vi "3.2.2_BOOST_Power_Tune.vi"(6 "Data in":T1, 8 "error in (no error)":errorcluster, 9 "AllControls In":T2, 10 "?":T3, 11 "Message Queue out":T4) -> (0 "error out":errorcluster, 1 "Flow":string, 2 "Data":T3, 3 "Message Queue Out":T4, 4 "Data out":T1)   [LabVIEW 2017]
uses:
  Depends/AMC/subVIs/TypeDefs/amc_Message Queue.ctl
  Depends/AMC/subVIs/TypeDefs/amc_Message.ctl
  Depends/Tools/Keyed Array/Tools_KeyedArray KeyedArray.ctl
  Ctrls/Data.ctl
  Ctrls/CSV_Data.ctl
  Ctrls/AllControls.ctl
  DIPC 692 Daemon API/typdef/get_parameter.ctl
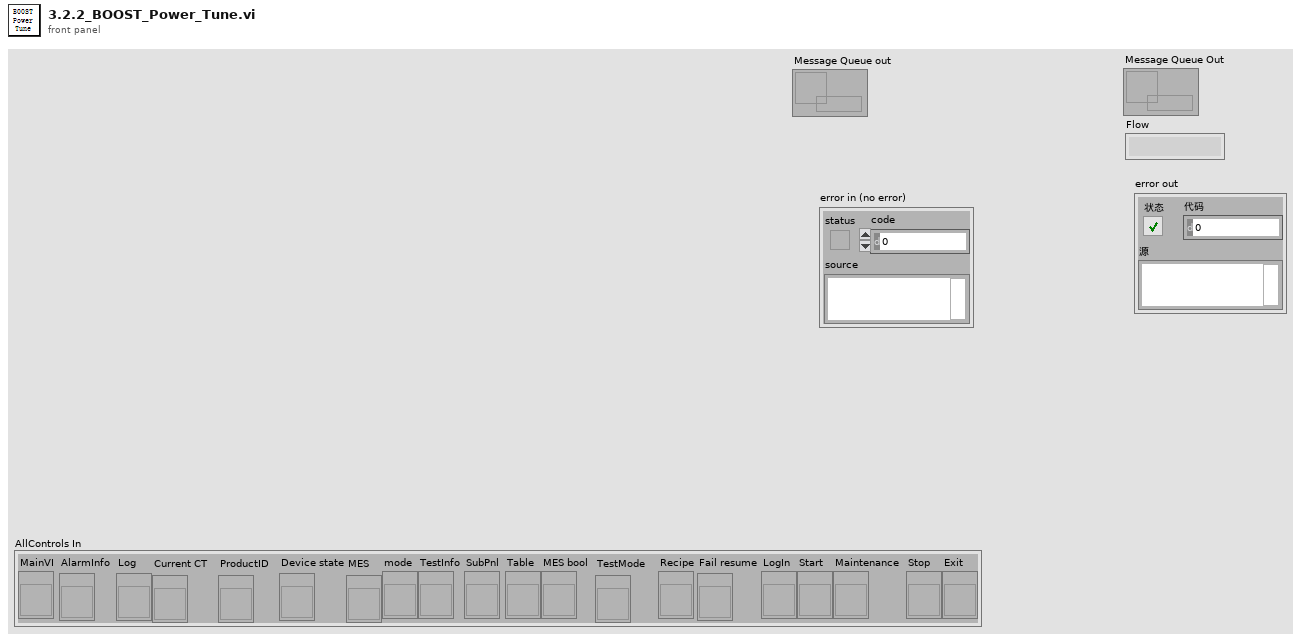
[diagram p1: front panel]
types:
  T1 = typedef "CSV_Data.ctl" = cluster{"Initialisation":cluster{"LMT - Connect UUT (con COM)":string, "LMT - Software Version (rrel)":string, "LMT - Write SKU file (wskuc)":string, "LMT - SKU file name":string, "Connect UUT DDM":string, "Read DDM EOL Timestamp - Mode":string, "Read DDM EOL Timestamp - Timestamp":string, "Read DDM EOL Timestamp - Rig ID":string, "Read DDM EOL Timestamp - Passmark ID":string, "Read DDM EOL Timestamp - Passmark Rev":string, "Software Version before flashing":string, "Read Hardware Serial":string, "UUT DDM SN":string, "Compare DDM SN with MES SN":string, "Backup PCBA Calibration EEPROM Response - CAL":string, "Flash Firmware Version":string, "Check SW Version":string, "Read DDM SW Version after flashing":string, "Set SKU Config":string, "Ready Status":string, "Set Device Mode to EOL":string, "DDM Parameter - Voltage":string, "DDM Parameter - Current":string, "DDM Parameter - Power":string, "DDM Parameter - Speed":string, "DDM Parameter - Pressure":string, "Tester Parameter - Voltage":string, "Tester Parameter - Current":string, "Tester Parameter - Power":string, "Tester Parameter - Ambient Pressure":string, "Tester Parameter - Ambient Temperature":string, "Calculated Parameter - DDM Pressure Corrected":string, "Calculated Parameter - DDM Real Power":string, "Calculated Parameter - Delta V":string}, "BEMF_Calibration":cluster{"Calibration Result - eol_cold_bemf_temp":string, "DDM Ambient Temp":string, "Restriction Plate Diameter":string, "Calibration Result - eol_bemf_mp_cold_coef_a":string, "Calibration Result - eol_bemf_mp_cold_coef_b":string, "Calibration Result - eol_bemf_mp_cold_coef_c":string, "Calibration Result - eol_bemf_lsi_cold_ref_coeffs":string, "Get - Calibration Result - eol_bemf_lsi_speed":string, "Get - Calibration Result - eol_bemf_lsi_integral_0":string, "Calibration Result - eol_bemf_lsi_integral_1":string, "Get - Calibration Result - eol_bemf_lsi_integral_2":string, "Get - Calibration Result - eol_cold_bemf":string, "Get - Calibration Result - eol_cold_bemf_fisf":string, "Finalise Calibration":string, "Compare -Calibration Result - eol_cold_bemf":string, "Compare -Calibration Result - eol_cold_bemf_fisf":string}, "ECO":cluster{"Reset Power Tune":string, "Reset BEMF FISF Calibration":string, "Restriction Plate Diameter":string, "ECO - Stabilisation Time":string, "ECO - DDM Parameter - Voltage":string, "ECO - DDM Parameter - Current":string, "ECO - DDM Parameter - Power":string, "ECO - DDM Parameter - Measured Power":string, "ECO - DDM Parameter - Speed":string, "ECO - DDM Parameter - Pressure":string, "ECO - Tester Parameter - Voltage":string, "ECO - Tester Parameter - Current":string, "ECO - Tester Parameter - Power":string, "ECO - Tester Parameter - Ambient Pressure":string, "ECO - Tester Parameter - Ambient Temperature":string, "ECO - Tester Parameter - Ambient Humidity":string, "ECO - Calculated Parameter - DDM Pressure Corrected":string, "ECO - Calculated Parameter - DDM Real Power":string, "ECO - Calculated Parameter - Delta V":string, "ECO - Calculated Parameter - Flowrate":string, "ECO - Calculated Parameter - Airwatt":string, "ECO - Formula":string, "PT ECO - Power Tune Mode Status":string}, "BOOST":cluster{"Restriction Plate Diameter":string, "BOOST - Stabilisation Time":string, "BOOST - DDM Parameter - Voltage":string, "BOOST - DDM Parameter - Current":string, "BOOST - DDM Parameter - Power":string, "BOOST - DDM Parameter - Measured Power":string, "BOOST - DDM Parameter - Speed":string, "BOOST - DDM Parameter - Pressure":string, "BOOST - Tester Parameter - Voltage":string, "BOOST - Tester Parameter - Current":string, "BOOST - Tester Parameter - Power":string, "BOOST - Tester Parameter - Ambient Pressure":string, "BOOST - Tester Parameter - Ambient Temperature":string, "BOOST - Tester Parameter - Ambient Humidity":string, "BOOST - Calculated Parameter - DDM Pressure Corrected":string, "BOOST - Calculated Parameter - DDM Real Power":string, "BOOST - Calculated Parameter - Delta V":string, "BOOST - Calculated Parameter - Flowrate":string, "BOOST - Calculated Parameter - Airwatt":string, "BOOST - Get AM Presence":string, "Air Muscle Turn Off Status":string, "BOOST - Air Muscle Calculated Parameter - Airwatt B":string, "BOOST - Air Muscle Calculate Airwatt Delta":string, "PT BOOST - Power Tune Mode Status":string, "Finalise Calibration":string, "ECO - Get AW Calibration value":string, "BOOST - Get AW Calibration value":string}, "MAX":cluster{"Restriction Plate Diameter":string, "MAX - Stabilisation Time":string, "Get Average Delta Tmag (LSIdelta_FISFdelta_LSItmag_FISFtmag_IIRtmag)":string, "Get Average Delta Tmag FISF":string, "MAX - DDM Parameter - Voltage":string, "MAX - DDM Parameter - Current":string, "MAX - DDM Parameter - Power":string, "MAX - DDM Parameter - Measured Power":string, "MAX - DDM Parameter - Speed":string, "MAX - DDM Parameter - Pressure":string, "MAX - Tester Parameter - Voltage":string, "MAX - Tester Parameter - Current":string, "MAX - Tester Parameter - Power":string, "MAX - Tester Parameter - Ambient Pressure":string, "MAX - Tester Parameter - Ambient Temperature":string, "MAX - Tester Parameter - Ambient Humidity":string, "MAX - Calculated Parameter - DDM Pressure Corrected":string, "MAX - Calculated Parameter - DDM Real Power":string, "MAX - Calculated Parameter - Delta V":string, "MAX - Calculated Parameter - Flowrate":string, "MAX - Calculated Parameter - Airwatt":string, "MAX_FISF_Check_Average_Delta_Tmag":string, "MAX - FISF - BEMF Finetune Result":string, "MAX tune - Delta P1":string, "MAX tune - Calculated Parameter - Airwatt":string, "Calculate Delta Airwatts - MAX finetune - Delta P2":string, "MAX finetune - DDM Parameter - Voltage":string, "MAX finetune - DDM Parameter - Current":string, "MAX finetune - DDM Parameter - Power":string, "MAX finetune - DDM Parameter - Measured Power":string, "MAX finetune - DDM Parameter - Speed":string, "MAX finetune - DDM Parameter - Pressure":string, "MAX finetune - Tester Parameter - Voltage":string, "MAX finetune - Tester Parameter - Current":string, "MAX finetune - Tester Parameter - Power":string, "MAX finetune - Tester Parameter - Ambient Pressure":string, "MAX finetune - Tester Parameter - Ambient Temperature":string, "MAX finetune - Tester Parameter - Ambient Humidity":string, "MAX finetune - Calculated Parameter - DDM Pressure Corrected":string, "MAX finetune - Calculated Parameter - DDM Real Power":string, "MAX finetune - Calculated Parameter - Delta V":string, "MAX finetune - Calculated Parameter - Flowrate":string, "MAX finetune - Calculated Parameter - Airwatt":string, "Check Derate Result":string, "Delta Tmag FISF":string, "Get Hot BEMF Result":string, "Calculate delta Pressure":string, "Finalise Calibration":string, "Calculate & Check Delta BEMF":string, "Delta P Airwatts Value":string}, "LL":cluster{"DDM Ambient Temp":string, "Restriction Plate Diameter":string, "LL - DDM Parameter - Voltage":string, "LL - DDM Parameter - Current":string, "LL - DDM Parameter - Power":string, "LL - DDM Parameter - Measured Power":string, "LL - DDM Parameter - Speed":string, "LL - DDM Parameter - Pressure":string, "LL - Tester Parameter - Voltage":string, "LL - Tester Parameter - Current":string, "LL - Tester Parameter - Power":string, "LL - DDM Real Power":string, "LL - Calibrate Task Detect LL":string}, "HL":cluster{"HL - DDM Parameter - Voltage":string, "HL - DDM Parameter - Current":string, "HL - DDM Parameter - Power":string, "HL - DDM Parameter - Measured Power":string, "HL - DDM Parameter - Speed":string, "HL - DDM Parameter - Pressure":string, "HL - Tester Parameter - Voltage":string, "HL - Tester Parameter - Current":string, "HL - Tester Parameter - Power":string, "HL - DDM Real Power":string, "HL - Calibrate Task Detect HL":string}, "LH":cluster{"Restriction Plate Diameter":string, "LH - DDM Parameter - Voltage":string, "LH - DDM Parameter - Current":string, "LH - DDM Parameter - Power":string, "LH - DDM Parameter - Measured Power":string, "LH - DDM Parameter - Speed":string, "LH - DDM Parameter - Pressure":string, "LH - Tester Parameter - Voltage":string, "LH - Tester Parameter - Current":string, "LH - Tester Parameter - Power":string, "LH - DDM Real Power":string, "LH - Calibrate Task Detect LH":string}, "HH":cluster{"HH - DDM Parameter - Voltage":string, "HH - DDM Parameter - Current":string, "HH - DDM Parameter - Power":string, "HH - DDM Parameter - Measured Power":string, "HH - DDM Parameter - Speed":string, "HH - DDM Parameter - Pressure":string, "HH - Tester Parameter - Voltage":string, "HH - Tester Parameter - Current":string, "HH - Tester Parameter - Power":string, "HH - DDM Real Power":string, "HH - Calibrate Task Detect HH":string}, "Inlet Blockage Calibration":cluster{"Inlet Blockage Calibration - DDM Parameter - Voltage":string, "Inlet Blockage Calibration - DDM Parameter - Current":string, "Inlet Blockage Calibration - DDM Parameter - Power":string, "Inlet Blockage Calibration - DDM Parameter - Measured Power":string, "Inlet Blockage Calibration - DDM Parameter - Speed":string, "Inlet Blockage Calibration - DDM Parameter - Pressure":string, "Inlet Blockage Calibration - Tester Parameter - Voltage":string, "Inlet Blockage Calibration - Tester Parameter - Current":string, "Inlet Blockage Calibration - Tester Parameter - Power":string, "Inlet Blockage Calibration - DDM Real Power":string, "Calibration Inlet Blockage_E":string, "Finalise Calibration":string, "Get Task Detect LL":string, "Get Task Detect HL":string, "Get Task Detect LH":string, "Get Task Detect HH":string, "Calibration Inlet Blockage":string, "Calibration eol cold bemf temp":string}, "GOOD":cluster{"GOOD UNIT - Clear EEPROM Error Log":string, "GOOD UNIT - Write Product Timestamp - Mode":string, "GOOD UNIT - Write Product Timestamp - Timestamp":string, "GOOD UNIT - Write Product Timestamp - Rig ID":string, "GOOD UNIT - Write Product Timestamp - Passmark ID":string, "GOOD UNIT - Write Product Timestamp - Passmark Rev":string, "GOOD UNIT - Set Device Mode to PROD":string, "GOOD UNIT - Backup PCBA Calibration EEPROM Response":string, "GOOD UNIT - Check Security Bit":string, "GOOD UNIT - Set Calibration Lock":string, "GOOD UNIT - Get_Calibration_Lock":string, "GOOD UNIT - Disconnect UUT":string}, "NG":cluster{"NG UNIT - Read NVM Error":string, "NG UNIT - Set Device Mode to FCT":string, "NG UNIT - Backup PCBA Calibration EEPROM Response - CAL":string, "NG UNIT - Backup PCBA Calibration EEPROM Response - ERROR":string, "NG UNIT - Backup PCBA Calibration EEPROM Response - USAGE":string, "NG UNIT - Disconnect UUT":string}, "SN":string, "Table":string[][], "Count":cluster{"Total":i32, "OK":i32, "NG":i32, "Yield":dbl}, "Start Time":timestamp, "daemon reference":refnum<k5>, "CT":dbl, "Config":string[][], "OK/NG":bool, "Station ID":string, "MES DDM SN":string, "MES PCBA SN":string, "Retest":string, "Lux":string, "Initialisation_Status":cluster{"LMT - Connect UUT (con COM)":string, "LMT - Software Version (rrel)":string, "LMT - Write SKU file (wskuc)":string, "LMT - SKU file name":string, "Connect UUT DDM":string, "Read DDM EOL Timestamp - Mode":string, "Read DDM EOL Timestamp - Timestamp":string, "Read DDM EOL Timestamp - Rig ID":string, "Read DDM EOL Timestamp - Passmark ID":string, "Read DDM EOL Timestamp - Passmark Rev":string, "Software Version before flashing":string, "Read Hardware Serial":string, "UUT DDM SN":string, "Compare DDM SN with MES SN":string, "Backup PCBA Calibration EEPROM Response - CAL":string, "Flash Firmware Version":string, "Check SW Version":string, "Read DDM SW Version after flashing":string, "Set SKU Config":string, "Ready Status":string, "Set Device Mode to EOL":string, "DDM Parameter - Voltage":string, "DDM Parameter - Current":string, "DDM Parameter - Power":string, "DDM Parameter - Speed":string, "DDM Parameter - Pressure":string, "Tester Parameter - Voltage":string, "Tester Parameter - Current":string, "Tester Parameter - Power":string, "Tester Parameter - Ambient Pressure":string, "Tester Parameter - Ambient Temperature":string, "Calculated Parameter - DDM Pressure Corrected":string, "Calculated Parameter - DDM Real Power":string, "Calculated Parameter - Delta V":string}, "BEMF_Calibration_Status":cluster{"Calibration Result - eol_cold_bemf_temp":string, "DDM Ambient Temp":string, "Restriction Plate Diameter":string, "Calibration Result - eol_bemf_mp_cold_coef_a":string, "Calibration Result - eol_bemf_mp_cold_coef_b":string, "Calibration Result - eol_bemf_mp_cold_coef_c":string, "Calibration Result - eol_bemf_lsi_cold_ref_coeffs":string, "Get - Calibration Result - eol_bemf_lsi_speed":string, "Get - Calibration Result - eol_bemf_lsi_integral_0":string, "Calibration Result - eol_bemf_lsi_integral_1":string, "Get - Calibration Result - eol_bemf_lsi_integral_2":string, "Get - Calibration Result - eol_cold_bemf":string, "Get - Calibration Result - eol_cold_bemf_fisf":string, "Finalise Calibration":string, "Compare -Calibration Result - eol_cold_bemf":string, "Compare -Calibration Result - eol_cold_bemf_fisf":string}, "ECO_Status":cluster{"Reset Power Tune":string, "Reset BEMF FISF Calibration":string, "Restriction Plate Diameter":string, "ECO - Stabilisation Time":string, "ECO - DDM Parameter - Voltage":string, "ECO - DDM Parameter - Current":string, "ECO - DDM Parameter - Power":string, "ECO - DDM Parameter - Measured Power":string, "ECO - DDM Parameter - Speed":string, "ECO - DDM Parameter - Pressure":string, "ECO - Tester Parameter - Voltage":string, "ECO - Tester Parameter - Current":string, "ECO - Tester Parameter - Power":string, "ECO - Tester Parameter - Ambient Pressure":string, "ECO - Tester Parameter - Ambient Temperature":string, "ECO - Tester Parameter - Ambient Humidity":string, "ECO - Calculated Parameter - DDM Pressure Corrected":string, "ECO - Calculated Parameter - DDM Real Power":string, "ECO - Calculated Parameter - Delta V":string, "ECO - Calculated Parameter - Flowrate":string, "ECO - Calculated Parameter - Airwatt":string, "ECO - Formula":string, "PT ECO - Power Tune Mode Status":string}, "BOOST_Status":cluster{"Restriction Plate Diameter":string, "BOOST - Stabilisation Time":string, "BOOST - DDM Parameter - Voltage":string, "BOOST - DDM Parameter - Current":string, "BOOST - DDM Parameter - Power":string, "BOOST - DDM Parameter - Measured Power":string, "BOOST - DDM Parameter - Speed":string, "BOOST - DDM Parameter - Pressure":string, "BOOST - Tester Parameter - Voltage":string, "BOOST - Tester Parameter - Current":string, "BOOST - Tester Parameter - Power":string, "BOOST - Tester Parameter - Ambient Pressure":string, "BOOST - Tester Parameter - Ambient Temperature":string, "BOOST - Tester Parameter - Ambient Humidity":string, "BOOST - Calculated Parameter - DDM Pressure Corrected":string, "BOOST - Calculated Parameter - DDM Real Power":string, "BOOST - Calculated Parameter - Delta V":string, "BOOST - Calculated Parameter - Flowrate":string, "BOOST - Calculated Parameter - Airwatt":string, "BOOST - Get AM Presence":string, "Air Muscle Turn Off Status":string, "BOOST - Air Muscle Calculated Parameter - Airwatt B":string, "BOOST - Air Muscle Calculate Airwatt Delta":string, "PT BOOST - Power Tune Mode Status":string, "Finalise Calibration":string, "ECO - Get AW Calibration value":string, "BOOST - Get AW Calibration value":string}, "MAX_Status":cluster{"Restriction Plate Diameter":string, "MAX - Stabilisation Time":string, "Get Average Delta Tmag (LSIdelta_FISFdelta_LSItmag_FISFtmag_IIRtmag)":string, "Get Average Delta Tmag FISF":string, "MAX - DDM Parameter - Voltage":string, "MAX - DDM Parameter - Current":string, "MAX - DDM Parameter - Power":string, "MAX - DDM Parameter - Measured Power":string, "MAX - DDM Parameter - Speed":string, "MAX - DDM Parameter - Pressure":string, "MAX - Tester Parameter - Voltage":string, "MAX - Tester Parameter - Current":string, "MAX - Tester Parameter - Power":string, "MAX - Tester Parameter - Ambient Pressure":string, "MAX - Tester Parameter - Ambient Temperature":string, "MAX - Tester Parameter - Ambient Humidity":string, "MAX - Calculated Parameter - DDM Pressure Corrected":string, "MAX - Calculated Parameter - DDM Real Power":string, "MAX - Calculated Parameter - Delta V":string, "MAX - Calculated Parameter - Flowrate":string, "MAX - Calculated Parameter - Airwatt":string, "MAX_FISF_Check_Average_Delta_Tmag":string, "MAX - FISF - BEMF Finetune Result":string, "MAX tune - Delta P1":string, "MAX tune - Calculated Parameter - Airwatt":string, "Calculate Delta Airwatts - MAX finetune - Delta P2":string, "MAX finetune - DDM Parameter - Voltage":string, "MAX finetune - DDM Parameter - Current":string, "MAX finetune - DDM Parameter - Power":string, "MAX finetune - DDM Parameter - Measured Power":string, "MAX finetune - DDM Parameter - Speed":string, "MAX finetune - DDM Parameter - Pressure":string, "MAX finetune - Tester Parameter - Voltage":string, "MAX finetune - Tester Parameter - Current":string, "MAX finetune - Tester Parameter - Power":string, "MAX finetune - Tester Parameter - Ambient Pressure":string, "MAX finetune - Tester Parameter - Ambient Temperature":string, "MAX finetune - Tester Parameter - Ambient Humidity":string, "MAX finetune - Calculated Parameter - DDM Pressure Corrected":string, "MAX finetune - Calculated Parameter - DDM Real Power":string, "MAX finetune - Calculated Parameter - Delta V":string, "MAX finetune - Calculated Parameter - Flowrate":string, "MAX finetune - Calculated Parameter - Airwatt":string, "Check Derate Result":string, "Delta Tmag FISF":string, "Get Hot BEMF Result":string, "Calculate delta Pressure":string, "Finalise Calibration":string, "Calculate & Check Delta BEMF":string, "Delta P Airwatts Value":string}, "LL_Status":cluster{"DDM Ambient Temp":string, "Restriction Plate Diameter":string, "LL - DDM Parameter - Voltage":string, "LL - DDM Parameter - Current":string, "LL - DDM Parameter - Power":string, "LL - DDM Parameter - Measured Power":string, "LL - DDM Parameter - Speed":string, "LL - DDM Parameter - Pressure":string, "LL - Tester Parameter - Voltage":string, "LL - Tester Parameter - Current":string, "LL - Tester Parameter - Power":string, "LL - DDM Real Power":string, "LL - Calibrate Task Detect LL":string}, "HL_Status":cluster{"HL - DDM Parameter - Voltage":string, "HL - DDM Parameter - Current":string, "HL - DDM Parameter - Power":string, "HL - DDM Parameter - Measured Power":string, "HL - DDM Parameter - Speed":string, "HL - DDM Parameter - Pressure":string, "HL - Tester Parameter - Voltage":string, "HL - Tester Parameter - Current":string, "HL - Tester Parameter - Power":string, "HL - DDM Real Power":string, "HL - Calibrate Task Detect HL":string}, "LH_Status":cluster{"Restriction Plate Diameter":string, "LH - DDM Parameter - Voltage":string, "LH - DDM Parameter - Current":string, "LH - DDM Parameter - Power":string, "LH - DDM Parameter - Measured Power":string, "LH - DDM Parameter - Speed":string, "LH - DDM Parameter - Pressure":string, "LH - Tester Parameter - Voltage":string, "LH - Tester Parameter - Current":string, "LH - Tester Parameter - Power":string, "LH - DDM Real Power":string, "LH - Calibrate Task Detect LH":string}, "HH_Status":cluster{"HH - DDM Parameter - Voltage":string, "HH - DDM Parameter - Current":string, "HH - DDM Parameter - Power":string, "HH - DDM Parameter - Measured Power":string, "HH - DDM Parameter - Speed":string, "HH - DDM Parameter - Pressure":string, "HH - Tester Parameter - Voltage":string, "HH - Tester Parameter - Current":string, "HH - Tester Parameter - Power":string, "HH - DDM Real Power":string, "HH - Calibrate Task Detect HH":string}, "Inlet Blockage Calibration_Status":cluster{"Inlet Blockage Calibration - DDM Parameter - Voltage":string, "Inlet Blockage Calibration - DDM Parameter - Current":string, "Inlet Blockage Calibration - DDM Parameter - Power":string, "Inlet Blockage Calibration - DDM Parameter - Measured Power":string, "Inlet Blockage Calibration - DDM Parameter - Speed":string, "Inlet Blockage Calibration - DDM Parameter - Pressure":string, "Inlet Blockage Calibration - Tester Parameter - Voltage":string, "Inlet Blockage Calibration - Tester Parameter - Current":string, "Inlet Blockage Calibration - Tester Parameter - Power":string, "Inlet Blockage Calibration - DDM Real Power":string, "Calibration Inlet Blockage_E":string, "Finalise Calibration":string, "Get Task Detect LL":string, "Get Task Detect HL":string, "Get Task Detect LH":string, "Get Task Detect HH":string, "Calibration Inlet Blockage":string, "Calibration eol cold bemf temp":string}, "GOOD_Status":cluster{"GOOD UNIT - Clear EEPROM Error Log":string, "GOOD UNIT - Write Product Timestamp - Mode":string, "GOOD UNIT - Write Product Timestamp - Timestamp":string, "GOOD UNIT - Write Product Timestamp - Rig ID":string, "GOOD UNIT - Write Product Timestamp - Passmark ID":string, "GOOD UNIT - Write Product Timestamp - Passmark Rev":string, "GOOD UNIT - Set Device Mode to PROD":string, "GOOD UNIT - Backup PCBA Calibration EEPROM Response":string, "GOOD UNIT - Check Security Bit":string, "GOOD UNIT - Set Calibration Lock":string, "GOOD UNIT - Get_Calibration_Lock":string, "GOOD UNIT - Disconnect UUT":string}, "NG_Status":cluster{"NG UNIT - Read NVM Error":string, "NG UNIT - Set Device Mode to FCT":string, "NG UNIT - Backup PCBA Calibration EEPROM Response - CAL":string, "NG UNIT - Backup PCBA Calibration EEPROM Response - ERROR":string, "NG UNIT - Backup PCBA Calibration EEPROM Response - USAGE":string, "NG UNIT - Disconnect UUT":string}, "SKU":string, "Plate_Diameter":string, "Alarm":string}
  T2 = typedef "AllControls.ctl" = cluster{"MainVI":refnum<vi>, "AlarmInfo":refnum<vi>, "Log":refnum<vi>, "Current CT":refnum<vi>, "ProductID":refnum<vi>, "Device state":refnum<vi>, "MES":refnum<vi>, "mode":refnum<vi>, "TestInfo":refnum<vi>, "SubPnl":refnum<vi>, "Table":refnum<vi>, "MES bool":refnum<vi>, "TestMode":refnum<vi>, "Recipe":refnum<vi>, "Fail resume":refnum<vi>, "LogIn":refnum<vi>, "Start":refnum<vi>, "Maintenance":refnum<vi>, "Stop":refnum<vi>, "Exit":refnum<vi>}
  T3 = typedef "Data.ctl" = cluster{"Initialisation":cluster{"DDM_Parameter":dbl[], "DDM_Parameter_status":bool[], "Get_Tester_Parameter":dbl[], "Get_Tester_Parameter_status":bool[], "Cal_Tester_Parameter":dbl[], "Cal_Tester_Parameter_status":bool[], "sw_version_before_status":bool, "sw_version_after_status":bool, "Set_SKU_Config_With_LMT_status":bool, "FCT_timestamp_status":bool, "LMT_Connect_to_UUT_status":bool}, "BEMF_Calibration":cluster{"Read_ambient_temperature":dbl, "Calibration_Vaule":dbl[], "Calibration_Vaule _B":dbl[], "Calibration_Vaule_status":bool[], "Calibration_Vaule_B_status":bool[]}, "ECO":cluster{"DDM_Parameter":dbl[], "DDM_Parameter_status":bool[], "Get_Tester_Parameter":dbl[], "Get_Tester_Parameter_status":bool[], "Cal_Tester_Parameter":dbl[], "Cal_Tester_Parameter_status":bool[], "DDM_Parameter_after_power_tune":dbl[], "Get_Tester_Parameter_after_power_tune":dbl[], "Cal_Tester_Parameter_after_power_tune":dbl[], "Cal_Tester_Parameter_after_power_tune_status":bool[], "Delta_P":dbl}, "BOOST":cluster{"DDM_Parameter":dbl[], "DDM_Parameter_status":bool[], "Get_Tester_Parameter":dbl[], "Get_Tester_Parameter_status":bool[], "Cal_Tester_Parameter":dbl[], "Cal_Tester_Parameter_status":bool[], "DDM_Parameter_after_power_tune":dbl[], "Get_Tester_Parameter_after_power_tune":dbl[], "Cal_Tester_Parameter_after_power_tune":dbl[], "Cal_Tester_Parameter_after_power_tune_status":bool[], "airwatts_am_off":dbl, "AW_Delta_(AM_on_and_off)":dbl, "AW_Delta_(AM_on_and_off)_Status":bool, "Delta_P":dbl}, "MAX":cluster{"Average_Tmag_Data":cluster{"LSI Delta in degC":dbl, "FISF Delta in degc":dbl, "LSI Tmag in degC":dbl, "Fisf Tmag in degC":dbl, "IIR Tmag in degC":dbl}, "DDM_Parameter":dbl[], "DDM_Parameter_status":bool[], "Get_Tester_Parameter":dbl[], "Get_Tester_Parameter_status":bool[], "Cal_Tester_Parameter":dbl[], "BEMF_Finetune":cluster{"eol_bemf_mp_cold_coef_c":dbl, "eol_cold_bemf_fisf_offset":dbl}, "AW_Tune":cluster{"delta_P1":dbl, "delta_P_Setting":dbl}, "DDM_Parameter_after_Airwatts_Tune":dbl[], "Get_Tester_Parameter_after_Airwatts_Tune":dbl[], "Cal_Tester_Parameter_after_Airwatts_Tune":dbl[], "DDM_Parameter_after_Airwatts_Finetune":dbl[], "Get_Tester_Parameter_after_Airwatts_Finetune":dbl[], "Cal_Tester_Parameter_after_Airwatts_Finetune":dbl[], "AW_Finetune":cluster{"delta_P2":dbl, "delta_P_Setting":dbl}, "Delta_Tmag_after_tune":cluster{"LSI Delta in degC":dbl, "FISF Delta in degc":dbl, "LSI Tmag in degC":dbl, "Fisf Tmag in degC":dbl, "IIR Tmag in degC":dbl}, "Hot Bemf in mV":dbl, "DDM_Pressure":dbl, "Delta_Pressure":dbl, " Cold Bemf in mV":dbl, " delta Bemf":dbl, " delta p":dbl, "Delta_Pressure_status":bool, " delta Bemf_status":bool, "LSI Delta in degC_status":bool, "FISF Delta in degc_status":bool, "Max_check_derate_status_status":bool, "Average_All_data":dbl[][], "Average_Tmag_Data_status":bool[], "Average_Tmag_Data_after_tune_status":bool[], "Cal_Tester_Parameter_status":bool[], "Cal_Tester_Parameter_status_after_Airwatts_Tune":bool[], "Cal_Tester_Parameter_status_after_Airwatts_FineTune":bool[]}, "Task_Detect_Calib":cluster{"LL":cluster{"DDM_Parameter":dbl[], "DDM_Parameter_status":bool[], "Get_Tester_Parameter":dbl[], "Get_Tester_Parameter_status":bool[], "Set_task_detect_A":dbl, "Set_task_detect_A_Status":bool}, "HL":cluster{"DDM_Parameter":dbl[], "DDM_Parameter_status":bool[], "Get_Tester_Parameter":dbl[], "Get_Tester_Parameter_status":bool[], "Set_task_detect_B":dbl, "Set_task_detect_B_Status":bool}, "LH":cluster{"DDM_Parameter":dbl[], "DDM_Parameter_status":bool[], "Get_Tester_Parameter":dbl[], "Get_Tester_Parameter_status":bool[], "Set_task_detect_C":dbl, "Set_task_detect_C_Status":bool}, "HH":cluster{"DDM_Parameter":dbl[], "DDM_Parameter_status":bool[], "Get_Tester_Parameter":dbl[], "Get_Tester_Parameter_status":bool[], "Set_task_detect_D":dbl, "Read_and_check_calibration_Status":bool[], "Set_task_detect_D_Status":bool}, "Get_eol_inlet_blockage_E":dbl, "Calib_vaule":cluster{"Get_task_detect_LL":dbl, "Get_task_detect_HL":dbl, "Get_task_detect_LH":dbl, "Get_task_detect_HH":dbl, "eol_inlet_blockage":dbl, "eol_code_bemf_temp":dbl}, "calibrated temp":dbl, "Inlet_Blockage_Calibration":cluster{"DDM_Parameter":dbl[], "DDM_Parameter_status":bool[], "Get_Tester_Parameter":dbl[], "Get_Tester_Parameter_status":bool[]}, "Get_eol_inlet_blockage_E_Status":bool}, "good":cluster{"Write_Product_TS":cluster{"TIMESTAMP":i64, "RIG_ID":i64, "PASSMARK_ID":i64, "PASSMARK_REV":i64}, "Read_Product_TS":cluster{"TIMESTAMP":i64, "RIG_ID":i64, "PASSMARK_ID":i64, "PASSMARK_REV":i64}, "Good_Check_Secuity_Bit_Stauts":bool}}
  T4 = typedef "amc_Message Queue.ctl" = refnum<queue>
  T5 = typedef "HD Config.ctl" = cluster{" PC":cluster{"PC Address":u8[], "PC Port":i32}, "FCO":cluster{"COM":refnum<visa-resource-name>, "Baudrate":u32}, "DC Power ":cluster{"COM":refnum<visa-resource-name>, "Baudrate":u32}, "PW3336":cluster{"COM":refnum<visa-resource-name>, "Baudrate":u32}, "Lefoo":cluster{"COM":refnum<visa-resource-name>, "Baudrate":u32}, "Tempt&Hum":cluster{"COM":refnum<visa-resource-name>, "Baudrate":u32}, "DIPC":cluster{"COM":refnum<visa-resource-name>}, "Daemon":cluster{"IP Address":string, "Port":u16, "Retry":u16}, "NFC":cluster{"COM":refnum<visa-resource-name>, "Baudrate":u32}, "Fail_resume_mode":bool, "GRR":bool}
  T6 = typedef "get_parameter.ctl" = string
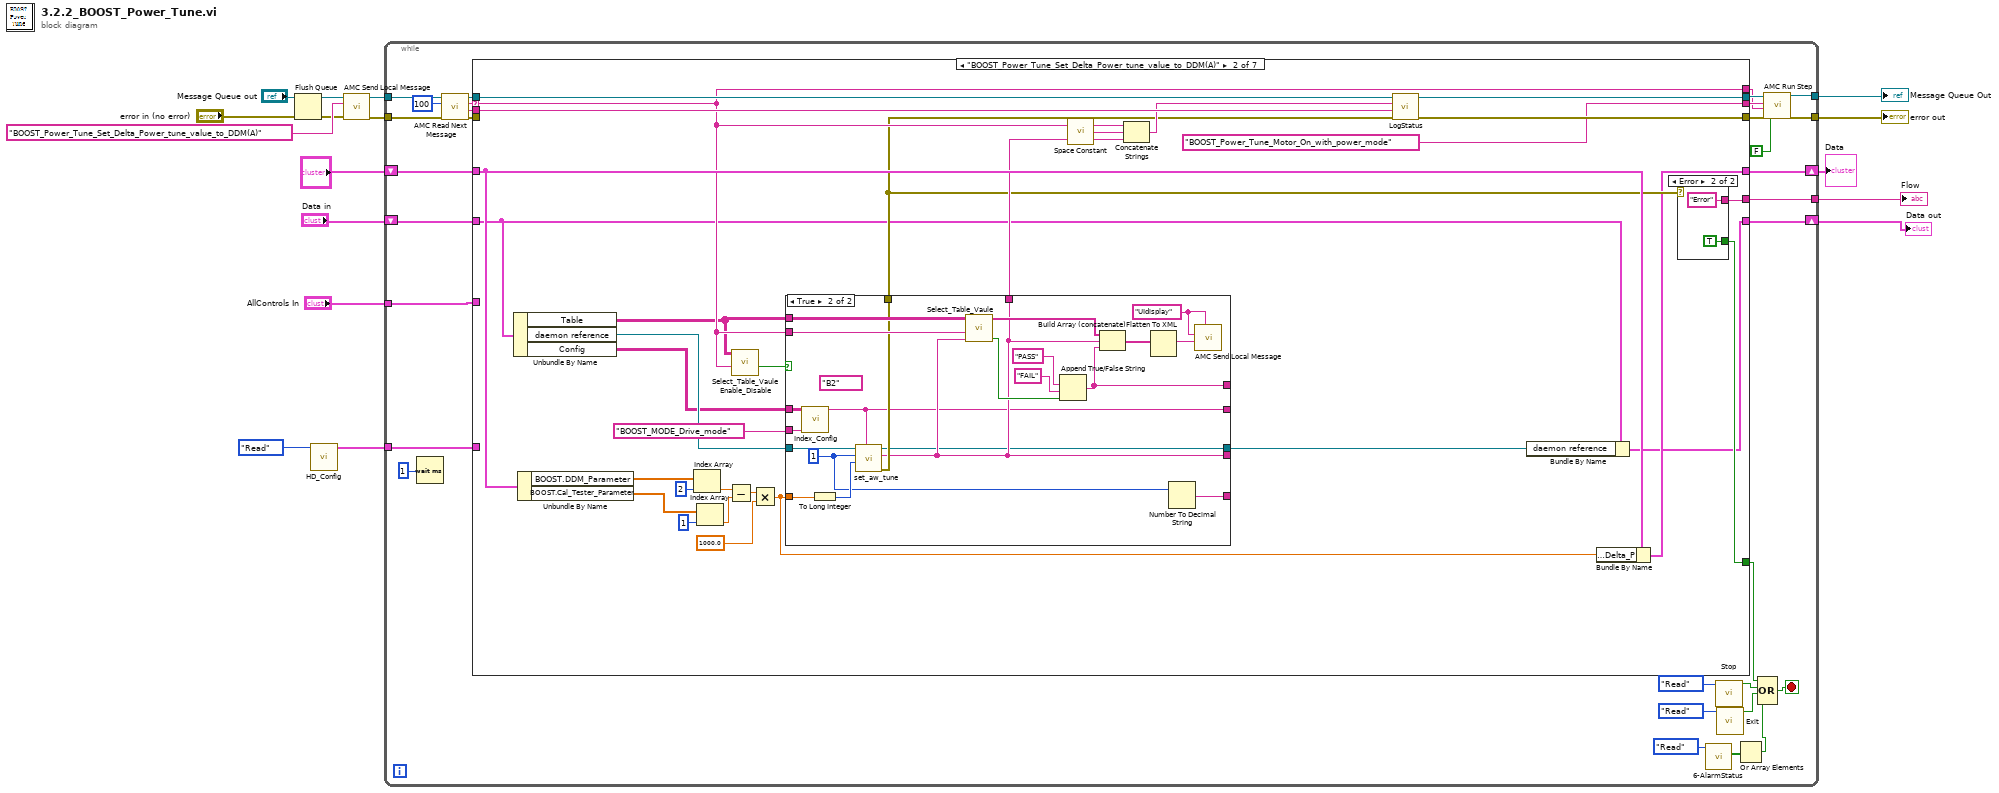
[diagram p0: block diagram]
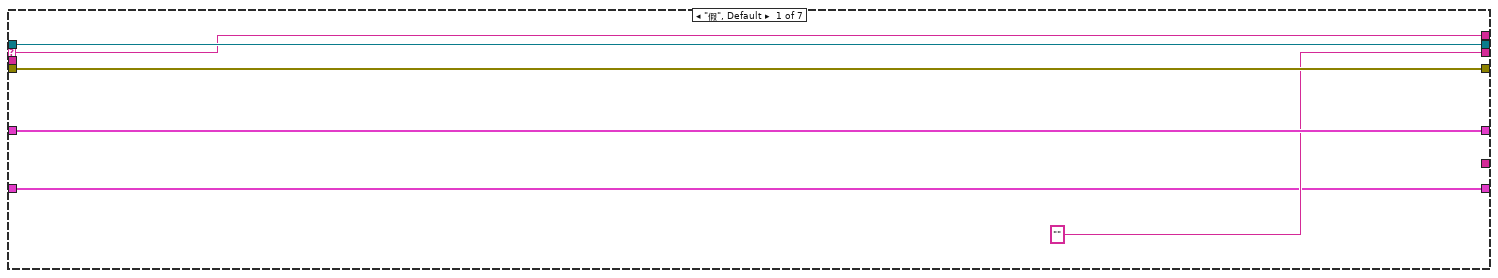
[diagram p2: hidden frame]
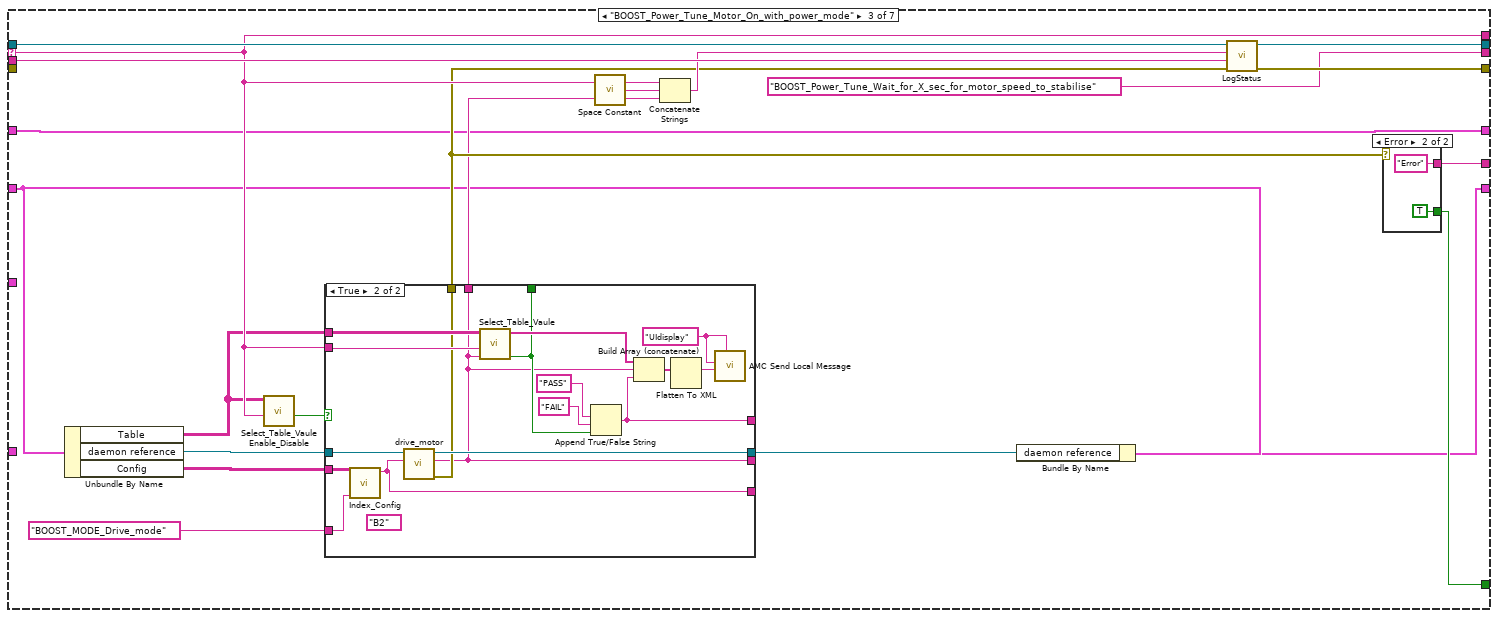
[diagram p5: hidden frame]
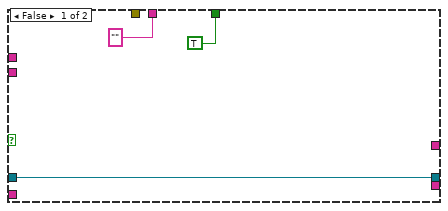
[diagram p7: hidden frame]
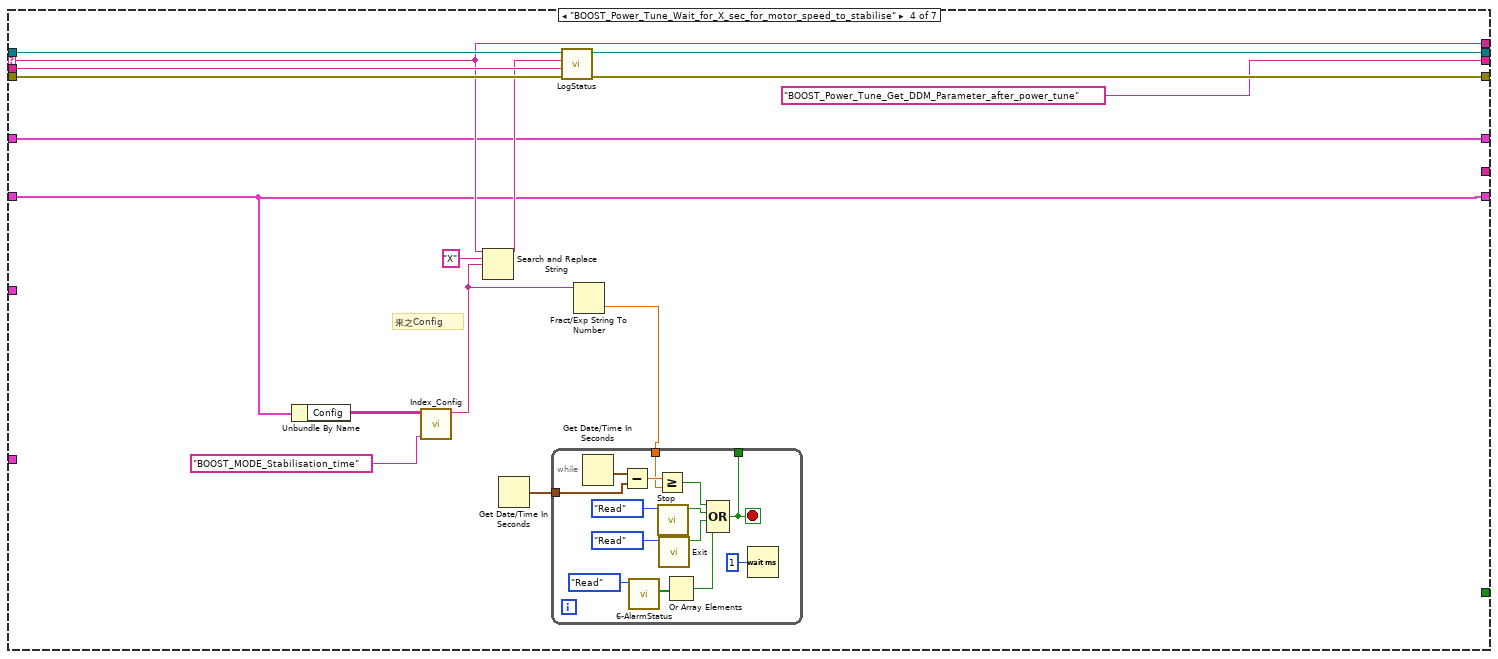
[diagram p8: hidden frame]
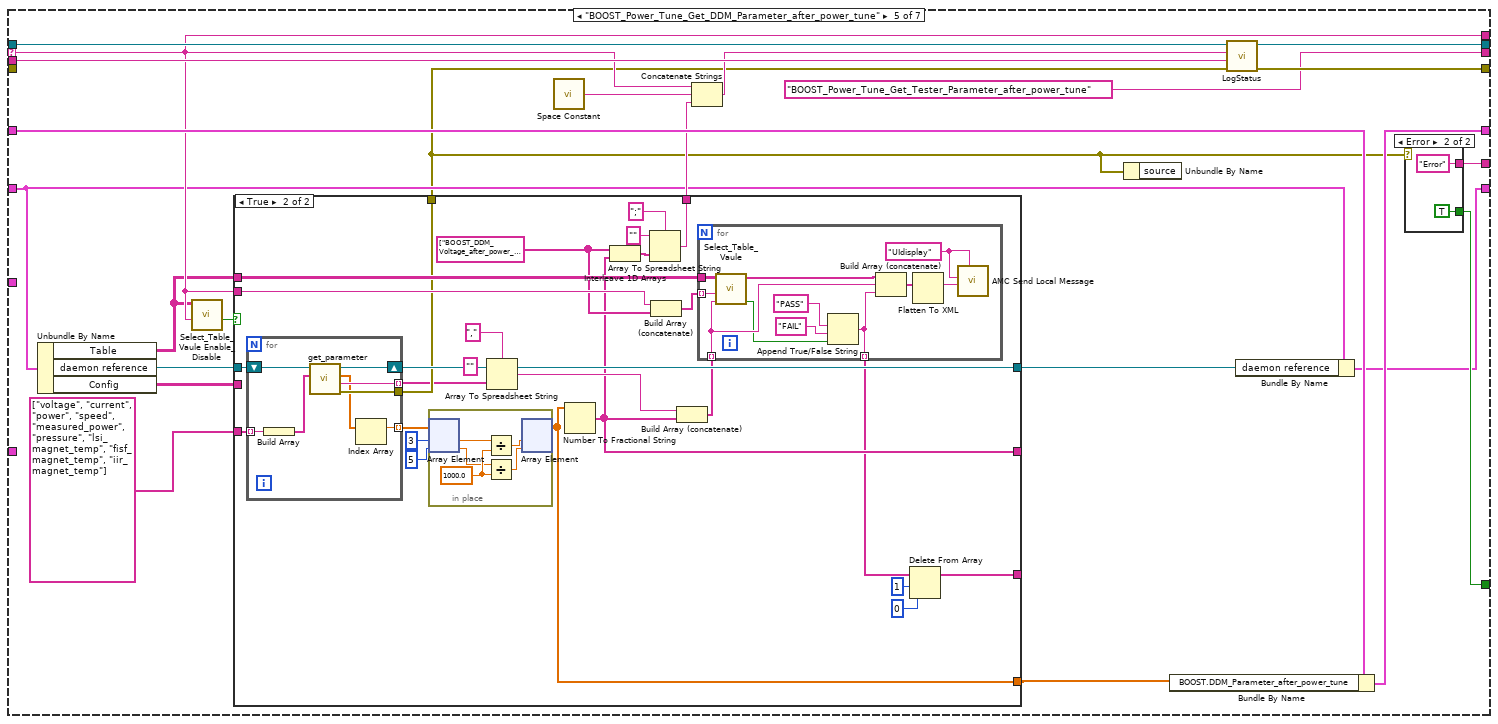
[diagram p9: hidden frame]
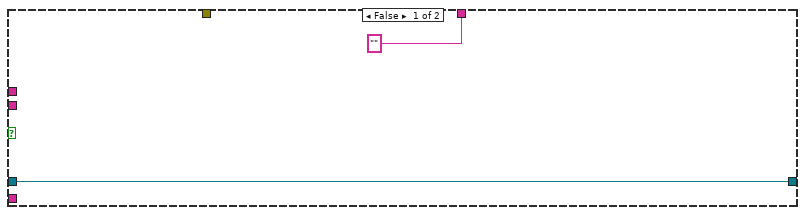
[diagram p11: hidden frame]
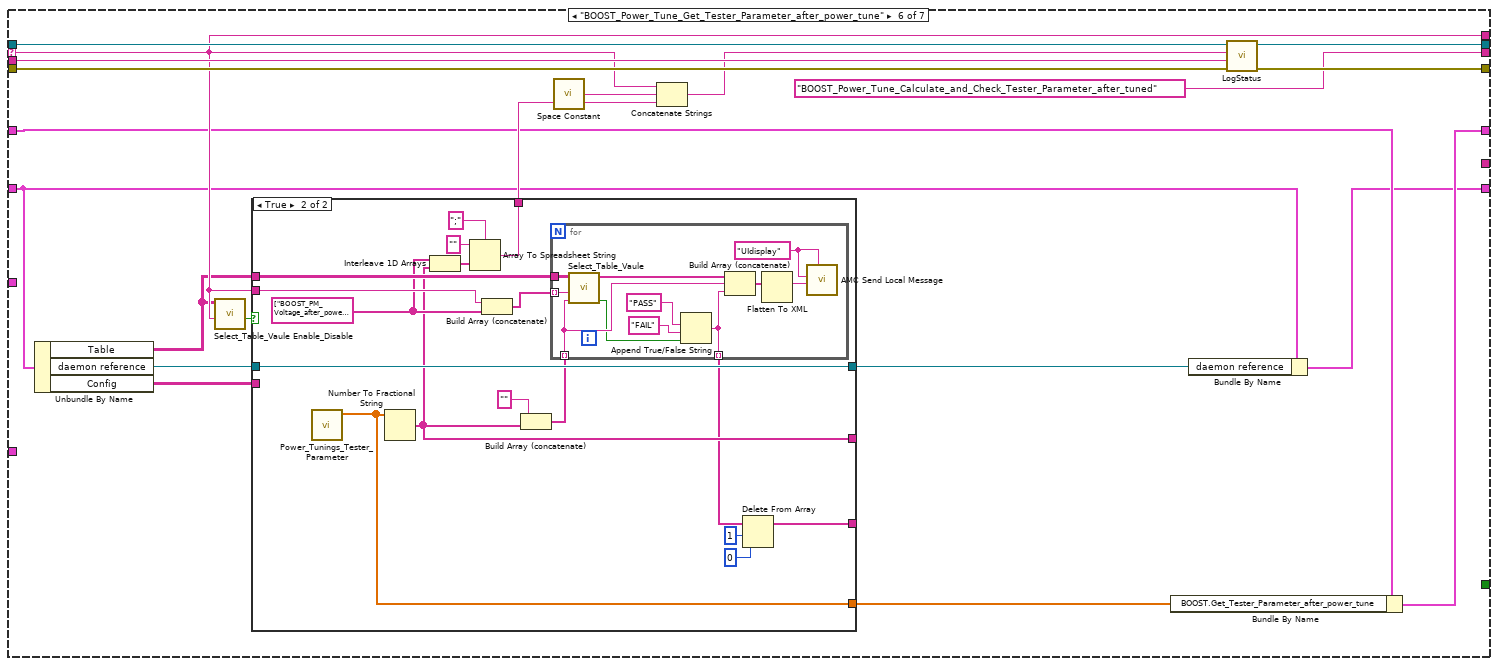
[diagram p12: hidden frame]
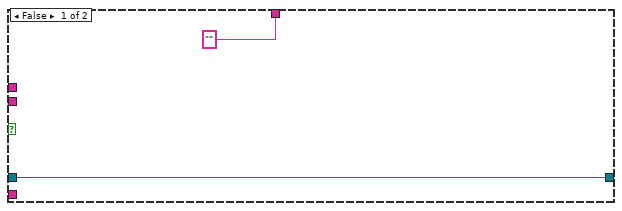
[diagram p13: hidden frame]
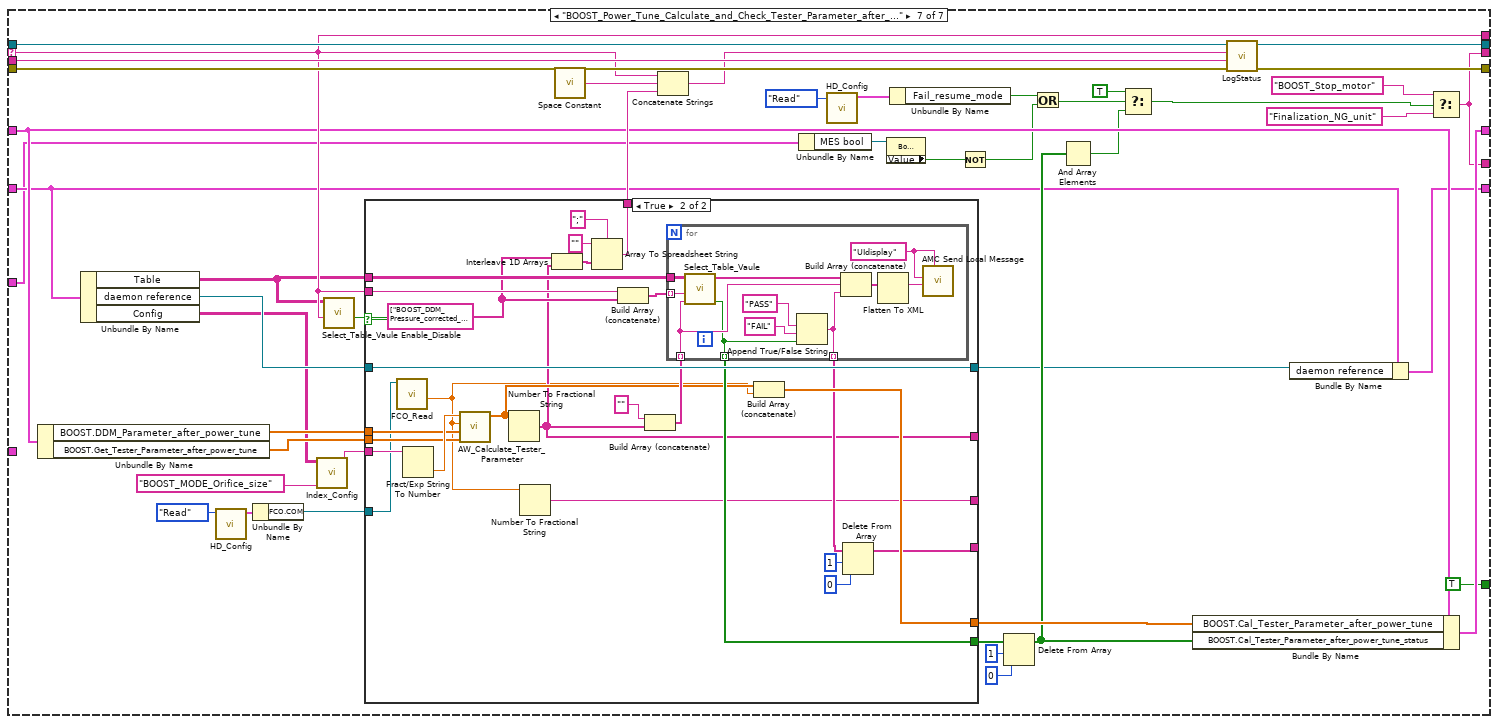
[diagram p14: hidden frame]
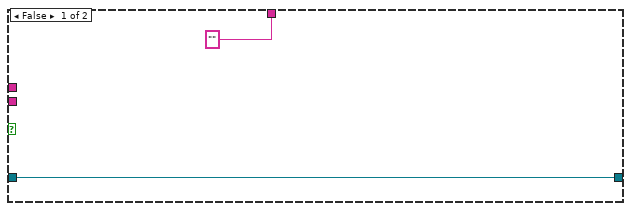
[diagram p15: hidden frame]
diagram:
  n1 = Flush Queue(queue="Message Queue out") -> (queue out=w4:T4)  [unwired: 1 in, 2 out]
  n2 = call "HD_Config.vi"("Step"=enum16{"Initial", "Write", "Read"}."Read") -> ("HD Config out"=w8:T5)  [unwired: 9 in, 1 out]
  n3 = call "AMC Send Local Message.vi"("error in (no error)"="error in (no error)", "Message Name"="BOOST_Power_Tune_Set_Delta_Power_tune_value_to_DDM(A)", "Message Queue in"=w4) -> ("error out"=w13:errorcluster, "Message Queue out"=w14:T4)  [unwired: 7 in]
  n4 = while {
    tunnel: w14 -> [w47]
    tunnel: [w43] -> w6
    tunnel: w13 -> [w41]
    tunnel: [w38] -> w5
    shift-right: [w34] -> w10
    shift-left: "?" -> [w35]
    tunnel: w8 -> [w33]
    tunnel: [w29] -> w7
    shift-right: [w20] -> w1
    shift-left: "Data in" -> [w22]
    tunnel: "AllControls In" -> [w21]
    stop <- w23 stop-if-true
    n5 = Wait (ms)(milliseconds to wait=u32 1 ("等待时间（毫秒）")) -> ()  [unwired: 1 out]
    n6 = call "AMC Read Next Message.vi"("error in (no error)"=w41, "timeout (1ms)"=100, "Message Queue in"=w47) -> ("error out"=w40:errorcluster, "Message Value"=w31:string, "Message Name"=w45:string, "Message Queue out"=w46:T4)  [unwired: 1 in, 4 out]
    n7 = case shown="\"BOOST_Power_Tune_Set_Delta_Power_tune_value_to_DDM(A)\"" w45 {
      selector: w45 -> [w50 w75 w120 w158 w191 w264 w339]
      tunnel: w46 -> [w53 w83 w127 w164 w200 w273 w347]
      tunnel: [w53 w83 w127 w164 w200 w273 w347] -> w44
      tunnel: w40 -> [w52 _ _ w163 _ w272 w346]
      tunnel: [w52 w82 w126 w162 w199 w271 w345] -> w39
      tunnel: [_ w63 w115 _ w184 _ TRUE] -> w24
      tunnel: w35 -> [w51 w79 w111 w154 w196 w260 w337]
      tunnel: [w51 w58 w111 w154 w195 w268 w343] -> w34
      tunnel: w31 -> [_ w81 w125 w161 w198 w270 w344]
      tunnel: [w50 w75 w120 w158 w191 w264 w339] -> w30
      tunnel: w33 -> [_ _ _ _ _ _ _]
      tunnel: ["" "BOOST_Power_Tune_Motor_On_with_power_mode" "BOOST_Power_Tune_Wait_for_X_sec_for_motor_speed_to_stabilise" "BOOST_Power_Tune_Get_DDM_Parameter_after_power_tune" "BOOST_Power_Tune_Get_Tester_Parameter_after_power_tune" "BOOST_Power_Tune_Calculate_and_Check_Tester_Parameter_after_tuned" w333] -> w32
      tunnel: [_ w64 w116 _ w185 _ w333] -> w29
      tunnel: w22 -> [w48 w57 w110 w150 w182 w257 w317]
      tunnel: w21 -> [_ _ _ _ _ _ w306]
      tunnel: [w48 w56 w108 w150 w179 w256 w316] -> w20
      frame "假", Default {
      }
      frame "BOOST_Power_Tune_Set_Delta_Power_tune_value_to_DDM(A)" {
        n8 = Unbundle By Name(w57) -> ("Table"=w61:string[][], "daemon reference"=w60:refnum<k5>, "Config"=w59:string[][])
        n9 = Unbundle By Name(w79) -> ("BOOST.DDM_Parameter"=w73:dbl[], "BOOST.Cal_Tester_Parameter"=w70:dbl[])
        n10 = Index Array(array=w73, index=2 ("索引")) -> (element=w69:dbl)
        n11 = Index Array(array=w70, index=1 ("索引")) -> (element=w68:dbl)
        n12 = Subtract(x=w69, y=w68) -> (x-y=w67:dbl)
        n13 = call "Select_Table_Vaule Enable_Disable.vi"("Action"=w75, "Table"=w61) -> ("Enable"=w74:bool)  [unwired: 8 in, 1 out]
        n14 = Multiply(x=w67, y=1000.0) -> (x*y=w55:dbl)
        n15 = case shown="True" w74 {
          tunnel: [_ w91] -> w76
          tunnel: w61 -> [_ w100]
          tunnel: w75 -> [_ w99]
          tunnel: w60 -> [w86 w98]
          tunnel: w59 -> [_ w95]
          tunnel: w55 -> [_ w96]
          tunnel: "BOOST_MODE_Drive_mode" -> [_ w94]
          tunnel: [_ w93] -> w62
          tunnel: [_ w92] -> _
          tunnel: [_ w91] -> _
          tunnel: [_ w89] -> _
          tunnel: [_ w88] -> _
          tunnel: [w86 w87] -> w54
          frame False {
          }
          frame True {
            w90 = 1 ("Index")
            (unwired) "B2" ("Power Mode or Target Power in W")
            w106 = "UIdisplay" ("Process (\"\" - local)")
            n16 = call "Index_Config.vi"("Action"=w94, "config"=w95) -> ("data"=w88:string)  [unwired: 9 in]
            n17 = To Long Integer(number=w96) -> (32bit integer=w97:i32)
            n18 = call "set_aw_tune.vi"("Power Mode or Target Power in W"=w88, "Offset Power mW"=w97, "Index"=w90, "daemon reference in"=w98) -> ("error out"=w93:errorcluster, "response"=w91:string, "daemon reference out"=w87:refnum<k5>)  [unwired: 4 in, 1 out]
            n19 = call "Select_Table_Vaule.vi"("Vaule"=w91, "Action"=w99, "Table"=w100) -> ("Result"=w101:bool, "vaule"=w107:string[])  [unwired: 7 in]
            n20 = Append True/False String(1:w101, 2:"FAIL" ("真字符串"), 3:"PASS" ("真字符串")) -> (0:w92:string)  [unwired: 1 in]
            n21 = Build Array (concatenate)(w107, w91, w92) -> (w105:string[])
            n22 = Flatten To XML(anything=w105) -> (xml string=w104:string)
            n23 = Number To Decimal String(number=w90) -> (decimal integer string=w89:string)  [unwired: 1 in]
            n24 = call "AMC Send Local Message.vi"("Process (\"\" - local)"=w106, "Message Value"=w104, "Message Name"=w106) -> ()  [unwired: 7 in, 2 out]
          }
        }
        n25 = call <vilib>:"Space Constant.vi"() -> ("String"=w77:string)
        n26 = Concatenate Strings(w75, w77, w76) -> (w78:string)
        n27 = call "LogStatus.vi"("error in (no error)"=w62, "last message"=w81, "message"=w78) -> ("error  out"=w82:errorcluster)  [unwired: 8 in]
        n28 = Bundle By Name(cluster=w57, "daemon reference"=w54) -> (w56:T1)
        n29 = Bundle By Name(cluster=w79, "BOOST.Delta_P"=w55) -> (w58:T3)
        n30 = case shown="Error" w62 {
          tunnel: [_ TRUE] -> w63
          tunnel: [_ "Error"] -> w64
          frame No Error {
          }
          frame Error {
          }
        }
      }
      frame "BOOST_Power_Tune_Motor_On_with_power_mode" {
        n31 = Unbundle By Name(w110) -> ("Table"=w119:string[][], "daemon reference"=w124:refnum<k5>, "Config"=w118:string[][])
        n32 = call "Select_Table_Vaule Enable_Disable.vi"("Action"=w120, "Table"=w119) -> ("Enable"=w121:bool)  [unwired: 8 in, 1 out]
        n33 = case shown="True" w121 {
          tunnel: w124 -> [w131 w149]
          tunnel: [TRUE w139] -> _
          tunnel: [w131 w143] -> w109
          tunnel: ["" ("response") w135] -> w113
          tunnel: w120 -> [_ w142]
          tunnel: w119 -> [_ w141]
          tunnel: w118 -> [_ w137]
          tunnel: [_ w138] -> w114
          tunnel: "BOOST_MODE_Drive_mode" -> [_ w136]
          tunnel: [_ w135] -> _
          tunnel: [_ w134] -> _
          tunnel: [_ w133] -> _
          frame False {
          }
          frame True {
            (unwired) "B2" ("Power Mode")
            w148 = "UIdisplay" ("Process (\"\" - local)")
            n34 = call "Index_Config.vi"("Action"=w136, "config"=w137) -> ("data"=w133:string)  [unwired: 9 in]
            n35 = call "drive_motor.vi"("Power Mode"=w133, "daemon reference in"=w149) -> ("error out"=w138:errorcluster, "response"=w135:string, "daemon reference out"=w143:refnum<k5>)  [unwired: 6 in, 1 out]
            n36 = call "Select_Table_Vaule.vi"("Vaule"=w135, "Action"=w142, "Table"=w141) -> ("Result"=w139:bool, "vaule"=w140:string[])  [unwired: 7 in]
            n37 = Append True/False String(1:w139, 2:"FAIL" ("真字符串"), 3:"PASS" ("真字符串")) -> (0:w134:string)  [unwired: 1 in]
            n38 = Build Array (concatenate)(w140, w135, w134) -> (w147:string[])
            n39 = Flatten To XML(anything=w147) -> (xml string=w146:string)
            n40 = call "AMC Send Local Message.vi"("Process (\"\" - local)"=w148, "Message Value"=w146, "Message Name"=w148) -> ()  [unwired: 7 in, 2 out]
          }
        }
        n41 = call <vilib>:"Space Constant.vi"() -> ("String"=w123:string)
        n42 = Concatenate Strings(w120, w123, w113) -> (w122:string)
        n43 = Bundle By Name(cluster=w110, "daemon reference"=w109) -> (w108:T1)
        n44 = call "LogStatus.vi"("error in (no error)"=w114, "last message"=w125, "message"=w122) -> ("error  out"=w126:errorcluster)  [unwired: 8 in]
        n45 = case shown="Error" w114 {
          tunnel: [_ TRUE] -> w115
          tunnel: [_ "Error"] -> w116
          frame No Error {
          }
          frame Error {
          }
        }
      }
      frame "BOOST_Power_Tune_Wait_for_X_sec_for_motor_speed_to_stabilise" {
        # "来之Config"
        n46 = Unbundle By Name(w150) -> ("Config"=w156:string[][])
        n47 = call "Index_Config.vi"("Action"="BOOST_MODE_Stabilisation_time", "config"=w156) -> ("data"=w153:string)  [unwired: 9 in]
        n48 = Search and Replace String(input string=w158, search string="X" ("搜索字符串"), replace string=w153) -> (result string=w157:string)  [unwired: 5 in, 3 out]
        n49 = Get Date/Time In Seconds() -> (seconds since 1Jan1904=w152:timestamp)
        n50 = call "LogStatus.vi"("error in (no error)"=w163, "last message"=w161, "message"=w157) -> ("error  out"=w162:errorcluster)  [unwired: 8 in]
        n51 = Fract/Exp String To Number(string=w153) -> (number=w151:dbl)  [unwired: 3 in, 1 out]
        n52 = while {
          tunnel: w152 -> [w171]
          tunnel: w151 -> [w168]
          tunnel: [w167] -> _
          stop <- w167 stop-if-true
          n53 = Get Date/Time In Seconds() -> (seconds since 1Jan1904=w172:timestamp)
          n54 = Subtract(x=w172, y=w171) -> (x-y=w170:dbl)
          n55 = call "6-AlarmStatus.vi"("Step"=enum16{"Initial", "Write", "Read"}."Read") -> ("AlarmValue Out"=w175:bool[])  [unwired: 9 in, 1 out]
          n56 = Greater Or Equal?(x=w170, y=w168) -> (x >= y?=w169:bool)
          n57 = call "Stop.vi"("Step"=enum16{"Initial", "Write", "Read"}."Read") -> ("Stop Out"=w173:bool)  [unwired: 9 in, 1 out]
          n58 = call "Exit.vi"("Step"=enum16{"Initial", "Write", "Read"}."Read" ("step")) -> ("Exit Out"=w177:bool)  [unwired: 9 in, 1 out]
          n59 = Or Array Elements(Boolean array=w175) -> (logical OR=w174:bool)
          n60 = Compound Arithmetic op=OR(w169, w173, w177, w174) -> (w167:bool)
          n61 = Wait (ms)(milliseconds to wait=u32 1 ("等待时间（毫秒）")) -> ()  [unwired: 1 out]
        }
      }
      frame "BOOST_Power_Tune_Get_DDM_Parameter_after_power_tune" {
        n62 = Unbundle By Name(w182) -> ("Table"=w190:string[][], "daemon reference"=w197:refnum<k5>, "Config"=w188:string[][])
        n63 = call "Select_Table_Vaule Enable_Disable.vi"("Action"=w191, "Table"=w190) -> ("Enable"=w189:bool)  [unwired: 8 in, 1 out]
        n64 = case shown="True" w189 {
          tunnel: w197 -> [w204 w229]
          tunnel: [w204 w228] -> w180
          tunnel: ["" ("software string") w221] -> w192
          tunnel: w191 -> [_ w226]
          tunnel: w190 -> [_ w230]
          tunnel: w188 -> [_ _]
          tunnel: [_ w216] -> w186
          tunnel: [_ w220] -> w181
          tunnel: T6[] ["voltage", "current", "power", "speed", "measured_power", "pressure", "lsi_magnet_temp", "fisf_magnet_temp", "iir_magnet_temp"] ("Parameter") -> [_ w214]
          tunnel: [_ w209] -> _
          tunnel: [_ w205] -> _
          frame False {
          }
          frame True {
            w215 = string[] ["BOOST_DDM_Voltage_after_power_tune", "BOOST_DDM_Current_after_power_tune", "BOOST_DDM_Power_after_power_tune", "BOOST_DDM_Speed_after_power_tune", "BOOST_DDM_Measured_Power_after_power_tune", "BOOST_DDM_Pressure_after_power_tune", "BOOST_lsi_magnet_temp_after_power_tune", "BOOST_fisf_magnet_temp_after_power_tune", "BOOST_iir_magnet_temp_after_power_tune"]
            n65 = for {
              tunnel: [w236] -> w213 mode=indexing
              tunnel: [w235] -> w220
              tunnel: [w231] -> w217 mode=indexing
              tunnel: w214 -> [w233] mode=indexing
              shift-right: [w237] -> w228
              shift-left: w229 -> [w238]
              n66 = Build Array(w233) -> (w232:T6[])
              n67 = call "get_parameter.vi"("Parameter"=w232, "daemon reference in"=w238) -> ("error out"=w235:errorcluster, "response"=w236:string, "values"=w234:dbl[], "daemon reference out"=w237:refnum<k5>)  [unwired: 5 in, 1 out]
              n68 = Index Array(array=w234) -> (element=w231:dbl)  [unwired: 1 in]
            }
            n69 = in-place {
              w243 = 1000.0
              n70 = in-place-array #1(w217, 3, 5) -> (w242:dbl, w239:dbl)
              n71 = Divide(x=w242, y=w243) -> (x/y=w241:dbl)
              n72 = Divide(x=w239, y=w243) -> (x/y=w240:dbl)
              n73 = in-place-array #1(w241, w240) -> (w216:dbl[])  [unwired: 2 out]
            }
            n74 = Array To Spreadsheet String(delimiter (Tab)=",", array=w213, 3:"" ("format string")) -> (spreadsheet string=w212:string)
            n75 = Number To Fractional String(number=w216) -> (F-format string=w209:string[])  [unwired: 3 in]
            n76 = Interleave 1D Arrays(w215, w209) -> (w222:string[])
            n77 = Array To Spreadsheet String(delimiter (Tab)=";" ("分隔符(Tab)"), array=w222, 3:"" ("格式字符串")) -> (spreadsheet string=w221:string)
            n78 = Build Array (concatenate)(w226, w215) -> (w227:string[])
            n79 = Build Array (concatenate)(w212, w209) -> (w225:string[])
            n80 = for {
              tunnel: w230 -> [w249]
              tunnel: w225 -> [w247] mode=indexing
              tunnel: w227 -> [w246] mode=indexing
              tunnel: [w244] -> w206 mode=indexing
              w254 = "UIdisplay" ("Process (\"\" - local)")
              n81 = call "Select_Table_Vaule.vi"("Vaule"=w247, "Action"=w246, "Table"=w249) -> ("Result"=w245:bool, "vaule"=w248:string[])  [unwired: 7 in]
              n82 = Append True/False String(1:w245, 2:"FAIL" ("真字符串"), 3:"PASS" ("真字符串")) -> (0:w244:string)  [unwired: 1 in]
              n83 = Build Array (concatenate)(w248, w247, w244) -> (w253:string[])
              n84 = Flatten To XML(anything=w253) -> (xml string=w252:string)
              n85 = call "AMC Send Local Message.vi"("Process (\"\" - local)"=w254, "Message Value"=w252, "Message Name"=w254) -> ()  [unwired: 7 in, 2 out]
            }
            n86 = Delete From Array(array=w206, length=1 ("长度"), index=0 ("索引")) -> (array with subset deleted=w205:string[])  [unwired: 1 out]
          }
        }
        n87 = call <vilib>:"Space Constant.vi"() -> ("String"=w194:string)
        n88 = Concatenate Strings(w191, w194, w192) -> (w193:string)
        n89 = Unbundle By Name(w181) -> ()  [unwired: 1 out]
        n90 = Bundle By Name(cluster=w196, "BOOST.DDM_Parameter_after_power_tune"=w186) -> (w195:T3)
        n91 = call "LogStatus.vi"("error in (no error)"=w181, "last message"=w198, "message"=w193) -> ("error  out"=w199:errorcluster)  [unwired: 8 in]
        n92 = Bundle By Name(cluster=w182, "daemon reference"=w180) -> (w179:T1)
        n93 = case shown="Error" w181 {
          tunnel: [_ TRUE] -> w184
          tunnel: [_ "Error"] -> w185
          frame No Error {
          }
          frame Error {
          }
        }
      }
      frame "BOOST_Power_Tune_Get_Tester_Parameter_after_power_tune" {
        n94 = Unbundle By Name(w257) -> ("Table"=w263:string[][], "daemon reference"=w269:refnum<k5>, "Config"=w261:string[][])
        n95 = call "Select_Table_Vaule Enable_Disable.vi"("Action"=w264, "Table"=w263) -> ("Enable"=w262:bool)  [unwired: 8 in, 1 out]
        n96 = case shown="True" w262 {
          tunnel: w269 -> [w275 w291]
          tunnel: [w275 w291] -> w255
          tunnel: ["" ("software string") w283] -> w265
          tunnel: w264 -> [_ w289]
          tunnel: w263 -> [_ w292]
          tunnel: w261 -> [_ _]
          tunnel: [_ w282] -> w258
          tunnel: [_ w280] -> _
          tunnel: [_ w276] -> _
          frame False {
          }
          frame True {
            w281 = string[] ["BOOST_PM_Voltage_after_power_tune", "BOOST_PM_Current_after_power_tune", "BOOST_PM_Power_after_power_tune", "BOOST_Ambient_Pressure_after_power_tune", "BOOST_Ambient_Temperature_after_power_tune", "BOOST_Ambient_humidity_after_power_tune", "BOOST_Tester_Reference_Ambient_Pressure_after_power_tune"]
            n97 = call "Power_Tunings_Tester_Parameter.vi"() -> ("Power_Tuning_Tester_Parameter"=w282:dbl[])  [unwired: 11 in]
            n98 = Number To Fractional String(number=w282) -> (F-format string=w280:string[])  [unwired: 3 in]
            n99 = Interleave 1D Arrays(w281, w280) -> (w284:string[])
            n100 = Array To Spreadsheet String(delimiter (Tab)=";" ("分隔符(Tab)"), array=w284, 3:"" ("格式字符串")) -> (spreadsheet string=w283:string)
            n101 = Build Array (concatenate)(w289, w281) -> (w290:string[])
            n102 = Build Array (concatenate)("", w280) -> (w288:string[])
            n103 = for {
              tunnel: w292 -> [w298]
              tunnel: w288 -> [w296] mode=indexing
              tunnel: w290 -> [w295] mode=indexing
              tunnel: [w293] -> w277 mode=indexing
              w303 = "UIdisplay" ("Process (\"\" - local)")
              n104 = call "Select_Table_Vaule.vi"("Vaule"=w296, "Action"=w295, "Table"=w298) -> ("Result"=w294:bool, "vaule"=w297:string[])  [unwired: 7 in]
              n105 = Append True/False String(1:w294, 2:"FAIL" ("真字符串"), 3:"PASS" ("真字符串")) -> (0:w293:string)  [unwired: 1 in]
              n106 = Build Array (concatenate)(w297, w296, w293) -> (w302:string[])
              n107 = Flatten To XML(anything=w302) -> (xml string=w301:string)
              n108 = call "AMC Send Local Message.vi"("Process (\"\" - local)"=w303, "Message Value"=w301, "Message Name"=w303) -> ()  [unwired: 7 in, 2 out]
            }
            n109 = Delete From Array(array=w277, length=1 ("长度"), index=0 ("索引")) -> (array with subset deleted=w276:string[])  [unwired: 1 out]
          }
        }
        n110 = call <vilib>:"Space Constant.vi"() -> ("String"=w267:string)
        n111 = Concatenate Strings(w264, w267, w265) -> (w266:string)
        n112 = Bundle By Name(cluster=w260, "BOOST.Get_Tester_Parameter_after_power_tune"=w258) -> (w268:T3)
        n113 = Bundle By Name(cluster=w257, "daemon reference"=w255) -> (w256:T1)
        n114 = call "LogStatus.vi"("error in (no error)"=w272, "last message"=w270, "message"=w266) -> ("error  out"=w271:errorcluster)  [unwired: 8 in]
      }
      frame "BOOST_Power_Tune_Calculate_and_Check_Tester_Parameter_after_tuned" {
        n115 = Unbundle By Name(w337) -> ("BOOST.DDM_Parameter_after_power_tune"=w323:dbl[], "BOOST.Get_Tester_Parameter_after_power_tune"=w322:dbl[])
        n116 = Unbundle By Name(w317) -> ("Table"=w320:string[][], "daemon reference"=w319:refnum<k5>, "Config"=w318:string[][])
        n117 = call "HD_Config.vi"("Step"=enum16{"Initial", "Write", "Read"}."Read") -> ("HD Config out"=w326:T5)  [unwired: 9 in, 1 out]
        n118 = Unbundle By Name(w326) -> ("FCO.COM"=w321:refnum<visa-resource-name>)
        n119 = call "Index_Config.vi"("Action"="BOOST_MODE_Orifice_size", "config"=w318) -> ("data"=w324:string)  [unwired: 9 in]
        n120 = call "Select_Table_Vaule Enable_Disable.vi"("Action"=w339, "Table"=w320) -> ("Enable"=w338:bool)  [unwired: 8 in, 1 out]
        n121 = case shown="True" w338 {
          tunnel: w319 -> [w349 w374]
          tunnel: [w349 w374] -> w315
          tunnel: ["" ("software string") w365] -> w340
          tunnel: w339 -> [_ w372]
          tunnel: w320 -> [_ w375]
          tunnel: [_ w357] -> w332
          tunnel: [_ w373] -> w331
          tunnel: w324 -> [_ w362]
          tunnel: w323 -> [_ w361]
          tunnel: w322 -> [_ w360]
          tunnel: w321 -> [_ w359]
          tunnel: [_ w353] -> _
          tunnel: [_ w352] -> _
          tunnel: [_ w350] -> _
          frame False {
          }
          frame True {
            w358 = string[] ["BOOST_DDM_Pressure_corrected_after_power_tune", "BOOST_DDM_Real_Power_after_power_tune", "BOOST_Delta_V_after_power_tune", "BOOST_Flow_rate_after_power_tune", "BOOST_AW_after_power_tune"]
            n122 = call "FCO_Read.vi"("VISA in"=w359) -> ("Pressure(Pa)"=w351:dbl)  [unwired: 7 in, 3 out]
            n123 = Fract/Exp String To Number(string=w362) -> (number=w364:dbl)  [unwired: 3 in, 1 out]
            n124 = call "AW_Calculate_Tester_Parameter.vi"("Tester Parameter"=w360, "DDM Parameter"=w361, "AW_Box_Pressure/Stag Total-Static Pressure rise"=w351, "Orifice_Plate_Diameter"=w364) -> ("Calculate Tester Parameter"=w363:dbl[])  [unwired: 7 in]
            n125 = Number To Fractional String(number=w363) -> (F-format string=w353:string[])  [unwired: 3 in]
            n126 = Number To Fractional String(number=w351) -> (F-format string=w350:string)  [unwired: 3 in]
            n127 = Interleave 1D Arrays(w358, w353) -> (w368:string[])
            n128 = Array To Spreadsheet String(delimiter (Tab)=";" ("分隔符(Tab)"), array=w368, 3:"" ("格式字符串")) -> (spreadsheet string=w365:string)
            n129 = Build Array (concatenate)(w372, w358) -> (w371:string[])
            n130 = Build Array (concatenate)("", w353) -> (w370:string[])
            n131 = for {
              tunnel: w375 -> [w381]
              tunnel: w370 -> [w379] mode=indexing
              tunnel: w371 -> [w378] mode=indexing
              tunnel: [w377] -> w373 mode=indexing
              tunnel: [w376] -> w354 mode=indexing
              w386 = "UIdisplay" ("Process (\"\" - local)")
              n132 = call "Select_Table_Vaule.vi"("Vaule"=w379, "Action"=w378, "Table"=w381) -> ("Result"=w377:bool, "vaule"=w380:string[])  [unwired: 7 in]
              n133 = Append True/False String(1:w377, 2:"FAIL" ("真字符串"), 3:"PASS" ("真字符串")) -> (0:w376:string)  [unwired: 1 in]
              n134 = Build Array (concatenate)(w380, w379, w376) -> (w385:string[])
              n135 = Flatten To XML(anything=w385) -> (xml string=w384:string)
              n136 = call "AMC Send Local Message.vi"("Process (\"\" - local)"=w386, "Message Value"=w384, "Message Name"=w386) -> ()  [unwired: 7 in, 2 out]
            }
            n137 = Build Array (concatenate)(w363, w351) -> (w357:dbl[])
            n138 = Delete From Array(array=w354, length=1 ("长度"), index=0 ("索引")) -> (array with subset deleted=w352:string[])  [unwired: 1 out]
          }
        }
        n139 = call <vilib>:"Space Constant.vi"() -> ("String"=w342:string)
        n140 = Concatenate Strings(w339, w342, w340) -> (w341:string)
        n141 = Unbundle By Name(w306) -> ("MES bool"=w313:refnum<vi>)
        n142 = call "HD_Config.vi"("Step"=enum16{"Initial", "Write", "Read"}."Read") -> ("HD Config out"=w314:T5)  [unwired: 9 in, 1 out]
        n143 = property class="Bool (严格)"(reference=w313) -> ("Value"=w311:bool)  [unwired: 1 in, 2 out]
        n144 = Unbundle By Name(w314) -> ("Fail_resume_mode"=w312:bool)
        n145 = Not(x=w311) -> (.not. x?=w309:bool)
        n146 = Delete From Array(array=w331, length=1 ("长度"), index=0 ("索引")) -> (array with subset deleted=w328:bool[])  [unwired: 1 out]
        n147 = Or(x=w312, y=w309) -> (x .or. y?=w310:bool)
        n148 = And Array Elements(Boolean array=w328) -> (logical AND=w305:bool)
        n149 = Select(t=TRUE, s=w310, f=w305) -> (s? t:f=w304:bool)
        n150 = Bundle By Name(cluster=w337, "BOOST.Cal_Tester_Parameter_after_power_tune"=w332, "BOOST.Cal_Tester_Parameter_after_power_tune_status"=w328) -> (w343:T3)
        n151 = call "LogStatus.vi"("error in (no error)"=w346, "last message"=w344, "message"=w341) -> ("error  out"=w345:errorcluster)  [unwired: 8 in]
        n152 = Bundle By Name(cluster=w317, "daemon reference"=w315) -> (w316:T1)
        n153 = Select(t="BOOST_Stop_motor", s=w304, f="Finalization_NG_unit") -> (s? t:f=w333:string)
      }
    }
    n154 = call "6-AlarmStatus.vi"("Step"=enum16{"Initial", "Write", "Read"}."Read") -> ("AlarmValue Out"=w18:bool[])  [unwired: 9 in, 1 out]
    n155 = call "Stop.vi"("Step"=enum16{"Initial", "Write", "Read"}."Read") -> ("Stop Out"=w26:bool)  [unwired: 9 in, 1 out]
    n156 = call "Exit.vi"("Step"=enum16{"Initial", "Write", "Read"}."Read" ("step")) -> ("Exit Out"=w25:bool)  [unwired: 9 in, 1 out]
    n157 = Or Array Elements(Boolean array=w18) -> (logical OR=w17:bool)
    n158 = Compound Arithmetic op=OR(w24, w26, w25, w17) -> (w23:bool)
    n159 = call "AMC Run Step.vi"("Message Queue In"=w44, "Message Name"=w32, "Message Value"=w30, "error in (no error)"=w39, "Mli/Sig"=FALSE) -> ("Message Queue Out"=w43:T4, "error out"=w38:errorcluster)  [unwired: 13 in]
  }
  "Message Queue Out" <- w6
  "error out" <- w5
  "Data" <- w10
  "Flow" <- w7
  "Data out" <- w1
